vi "test_VI Set_Get Protocol Error.vi"(8 "error in (no error)":errorcluster, 11 "TestCase in":refnum<class "Instrument Addon Scripting API Custom Device Unit Tests.lvclass">) -> (0 "error out":errorcluster, 3 "TestCase out":refnum<class "Instrument Addon Scripting API Custom Device Unit Tests.lvclass">)   [LabVIEW 2018, in "Instrument Addon Scripting API Custom Device Unit Tests.lvclass"]
uses:
  Instrument Addon Scripting API Custom Device Unit Tests.lvclass
  Addon/Support Libraries/Protocols.lvlibp/Protocol Parent/Protocol Parent.lvclass
  NationalInstruments.VeriStand.SystemDefinitionAPI
  Instrument Addon Scripting API Test Assets/Instrument Addon Scripting API Test Assets.lvclass
  <vilib>/addons/_JKI Toolkits/VI Tester/TestCase.llb/TestCase.lvclass
  APIs/Scripting API/Instrument Addon Scripting API.lvlib
  C:/Program Files (x86)/National Instruments/LabVIEW 2018/vi.lib/addons/_JKI Toolkits/VI Tester/TestCase.llb/TestCase.lvclass
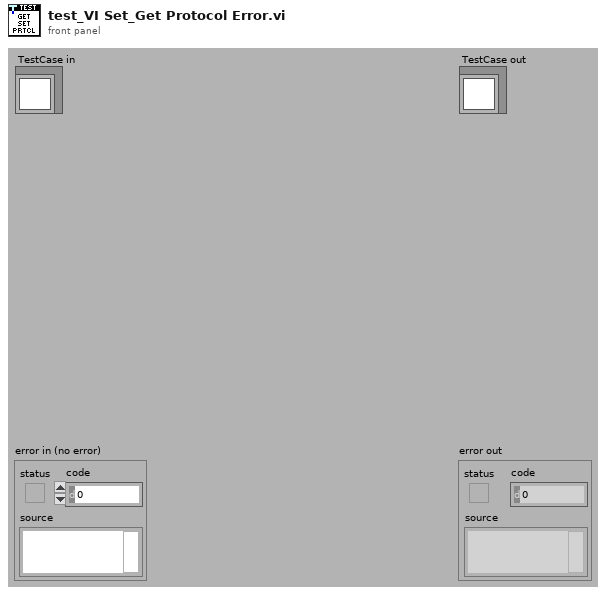
[diagram p1: front panel]
types:
  T1 = typedef "Custom Device API.lvlib/Custom Device Item Ref.ctl" = u64
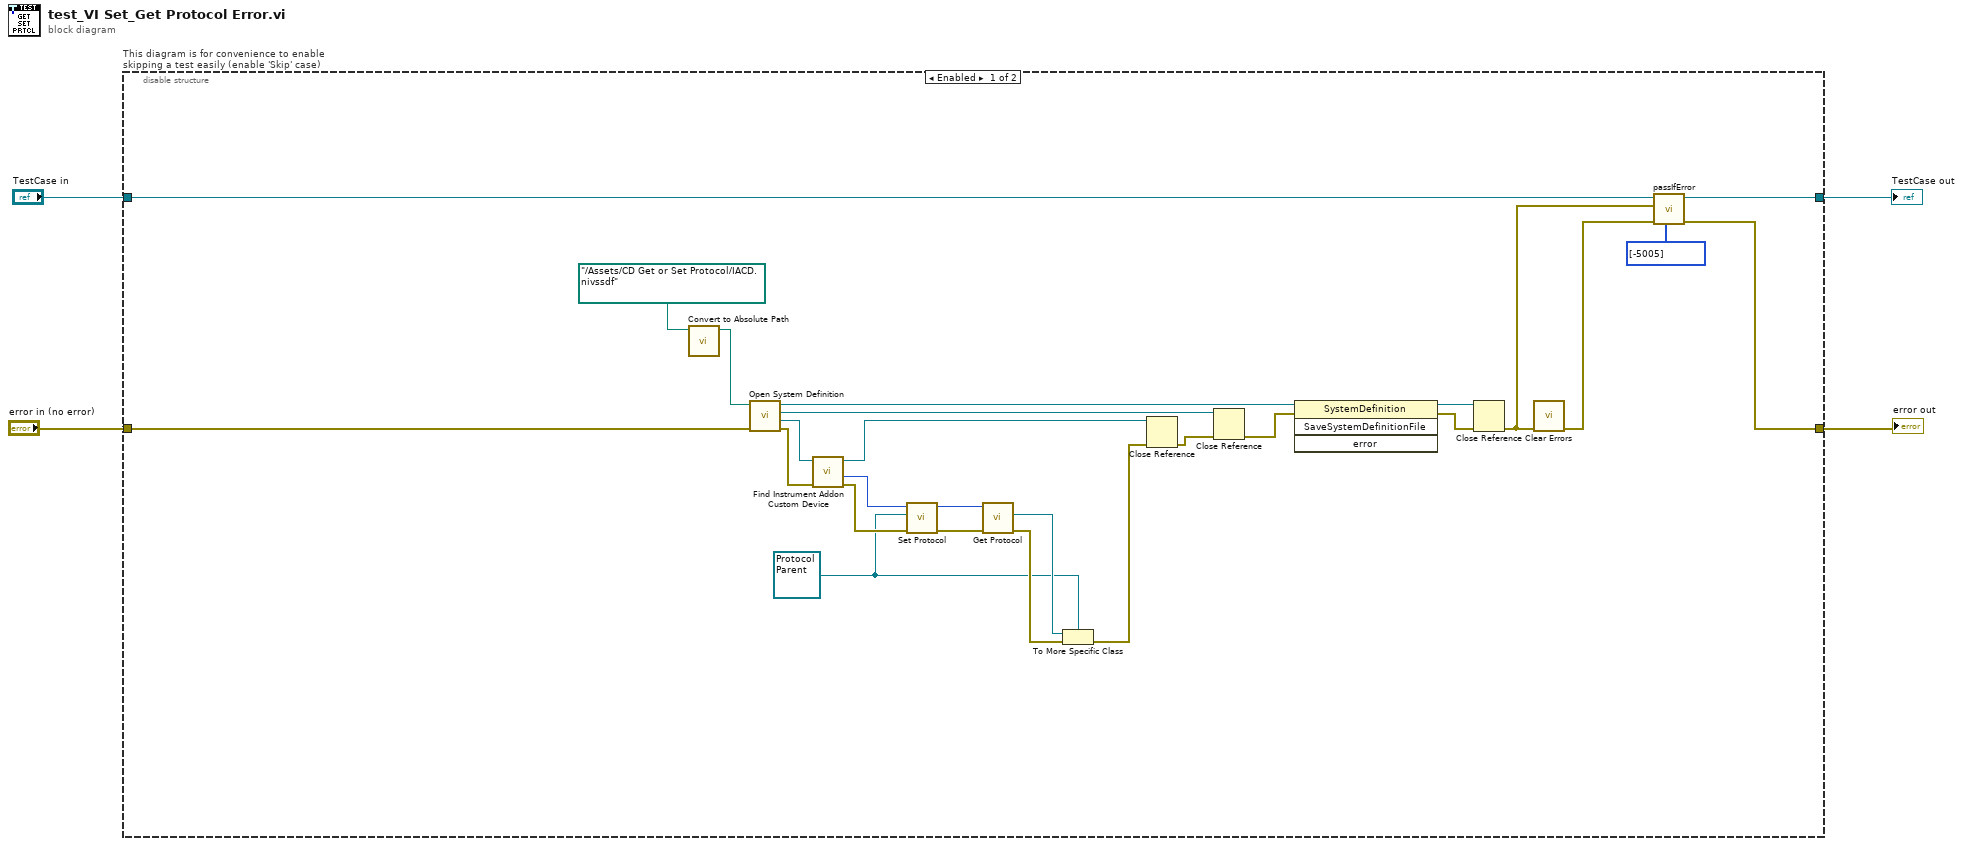
[diagram p0: block diagram]
diagram:
  n1 = disable-structure "This diagram is for convenience to enable skipping a test easily (enable 'Skip' case)" shown="Enabled" {
    disable-tunnel: "TestCase in" -> [w10 w34]
    disable-tunnel: [w9 w32] -> w1
    disable-tunnel: [w5 w33] -> w3
    disable-tunnel: "error in (no error)" -> [w30 w31]
    frame Enabled {
      w11 = refnum<class "Protocol Parent.lvclass"> refnum ("Protocols.lvlibp:Protocol Parent.lvclass")
      n2 = call "Convert to Absolute Path.vi"("System Definition File"=path "../Assets/CD Get or Set Protocol/IACD.nivssdf" ("SDF file")) -> ("Absolute Path"=w28:path)  [unwired: 10 in]
      n3 = call "Open System Definition.vi"("error in (no error)"=w30, "System Definition File"=w28) -> ("error out"=w25:errorcluster, "Target Refnum"=w24:refnum<k24>, "Root Refnum"=w27:refnum<k24>, "System Definition Refnum"=w18:refnum<k24>)  [unwired: 6 in]
      n4 = call "Find Instrument Addon Custom Device.vi"("error in"=w25, "target in"=w24) -> ("error out"=w23:errorcluster, "NodeID"=w22:u64, "target out"=w21:refnum<k24>)  [unwired: 7 in]
      n5 = call "Set Protocol.vi"("Error In"=w23, "Protocol in"=w11, "Instrument Addon Refnum In"=w22) -> ("Error Out"=w19:errorcluster, "Instrument Addon Refnum Out"=w20:T1)  [unwired: 7 in]
      n6 = call "Get Protocol.vi"("Error In"=w19, "Instrument Addon Refnum In"=w20) -> ("Error Out"=w13:errorcluster, "Protocol"=w14:refnum<class "Protocol Parent.lvclass">)  [unwired: 7 in, 1 out]
      n7 = To More Specific Class(target class=w11, reference=w14, error in=w13) -> (error out=w12:errorcluster)  [unwired: 1 out]
      n8 = Close Reference(reference=w21, error in (no error)=w12) -> (error out=w26:errorcluster)
      n9 = Close Reference(reference=w27, error in (no error)=w26) -> (error out=w17:errorcluster)
      n10 = invoke class="SystemDefinition" method="SaveSystemDefinitionFile"(reference=w18, error in=w17) -> (reference out=w16:refnum<k24>, error out=w15:errorcluster)  [unwired: 2 in, 2 out]
      n11 = Close Reference(reference=w16, error in (no error)=w15) -> (error out=w7:errorcluster)
      n12 = call <vilib>:"Clear Errors.vi"("error in (no error)"=w7) -> ("error out"=w6:errorcluster)  [unwired: 5 in, 1 out]
      n13 = call-dynamic "passIfError.vi"("passing error codes (default = any error code)"=i32[] [-5005], "error in (no error)"=w6, "error"=w7, "TestCase in"=w10) -> ("error out"=w5:errorcluster, "TestCase out"=w9:refnum<class "Instrument Addon Scripting API Custom Device Unit Tests.lvclass">)  [unwired: 6 in]
    }
    frame Disabled {
      # "skip test result while test is under development"
      n14 = call <vilib>:"skip.vi"("error in (no error)"=w31, "TestCase in"=w34) -> ("error out"=w33:errorcluster, "TestCase out"=w32:refnum<class "Instrument Addon Scripting API Custom Device Unit Tests.lvclass">)  [unwired: 8 in]
    }
  }
  "error out" <- w3
  "TestCase out" <- w1
